vi "StartCSMs.vi"(8 "error in":errorcluster, 11 "Array":T1(array[cluster])=[{"prototype"="Normal-CSM.vi", "name"="Normal", "num"=1, "index"=0}, {"prototype"="Normal-CSM.vi", "name"=".SysLevel", "num"=1, "index"=0}, {"prototype"="Normal-CSM.vi", "name"="Normal.SubModule", "num"=1, "index"=0}, {"prototype"="Normal-CSM.vi", "name"="Normal2", "num"=1, "index"=0}, {"prototype"="Normal-CSM.vi", "name"=".SysLevel2", "num"=1, "index"=0}, {"prototype"="Normal-CSM.vi", "name"="Normal.SubModule2", "num"=1, "index"=0}, {"prototype"="Normal-CSM.vi", "name"="worker", "num"=3, "index"=0}, {"prototype"="Normal-CSM.vi", "name"="worker2", "num"=3, "index"=0}, {"prototype"="Chain1.vi", "name"="Chain", "num"=1, "index"=1}, {"prototype"="Chain2.vi", "name"="Chain", "num"=1, "index"=2}, {"prototype"="Chain3.vi", "name"="Chain", "num"=1, "index"=3}, {"prototype"="CSM\\CSM-Testcase.lvlibp\\testcases\\CSM\\Normal-CSM.vi", "name"="lvlibp", "num"=1, "index"=0}, {"prototype"="CSM\\CSM-Testcase2.lvlibp\\testcases\\CSM\\Normal-CSM.vi", "name"="lvlibp2", "num"=1, "index"=0}]) -> (0 "error out":errorcluster, 2 "CSMs":string[](array[string]))   [LabVIEW 2017]
uses:
  src/user.lib/_NEVSTOP/Communicable State Machine(CSM)/Communicable State Machine.lvlib
  src/user.lib/_NEVSTOP/Communicable State Machine(CSM)/_Shared/CSM Shared.lvlib
panel:
  out "Waited (ms)":u32
  out "CSMs Left":string[](array[string])
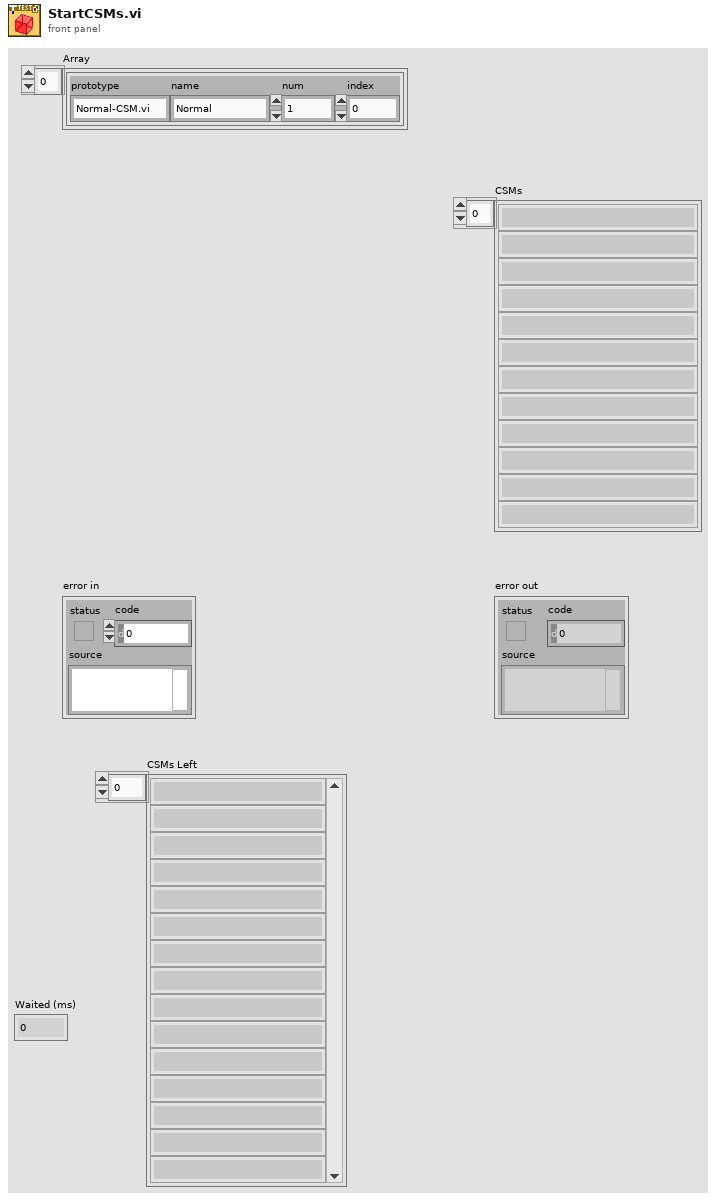
[diagram p1: front panel]
types:
  T1 = cluster{"prototype":string, "name":string, "num":i32, "index":i32}[]
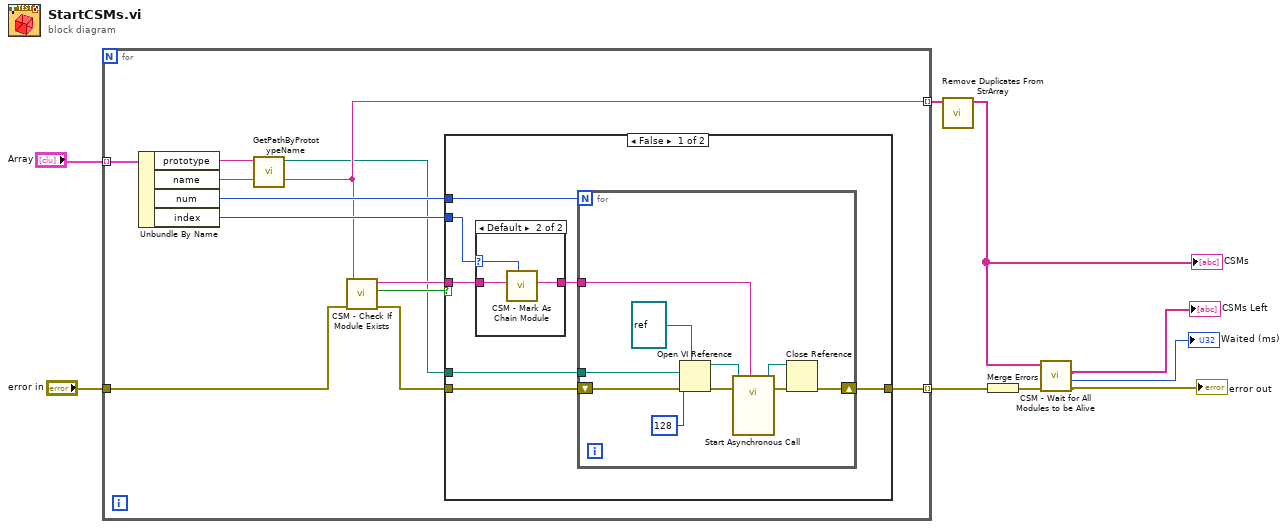
[diagram p0: block diagram]
diagram:
  n1 = for {
    tunnel: [w20] -> w6 mode=indexing
    tunnel: "Array" -> [w16] mode=indexing
    tunnel: "error in" -> [w15]
    tunnel: [w12] -> w7 mode=indexing
    n2 = Unbundle By Name(w16) -> ("prototype"=w11:string, "name"=w12:string, "num"=w14:i32, "index"=w13:i32)
    n3 = call "GetPathByPrototypeName.vi"("prototype"=w11) -> ("path"=w10:path)  [unwired: 10 in]
    n4 = call "CSM - Check If Module Exists.vi"("Error In"=w15, "CSM Name"=w12) -> ("error out"=w19:errorcluster, "Exist?"=w17:bool, "CSM Name (Dup)"=w18:string)  [unwired: 7 in]
    n5 = case shown="False" w17 {
      tunnel: [w27 w42] -> w20
      tunnel: w19 -> [w26 w42]
      tunnel: w18 -> [w23 _]
      tunnel: w14 -> [w25 _]
      tunnel: w13 -> [w24 _]
      tunnel: w10 -> [w21 _]
      frame False {
        n6 = case shown="Default" w24 {
          selector: w24 -> [_ w31]
          tunnel: w23 -> [w28 w30]
          tunnel: [w28 w29] -> w22
          frame 0 {
          }
          frame Default {
            n7 = call "CSM - Mark As Chain Module.vi"("Order"=w31, "CSM Name"=w30) -> ("CSM Name (Marked As Chain)"=w29:string)  [unwired: 8 in]
          }
        }
        n8 = for {
          N: w25 -> [_]
          tunnel: w22 -> [w35]
          shift-right: [w36] -> w27
          shift-left: w26 -> [w33]
          tunnel: w21 -> [w32]
          n9 = Open VI Reference(type specifier VI Refnum (for type only)=refnum<vi> refnum, vi path=w32, options=128, error in (no error)=w33) -> (vi reference=w38:refnum<vi>, error out=w40:errorcluster)  [unwired: 2 in]
          n10 = call-by-ref "Start Asynchronous Call"(reference=w38, error in=w40, "Name (\"\" to Use UUID)"=w35) -> (reference out=w37:refnum<vi>, error out=w39:errorcluster)  [unwired: 11 in]
          n11 = Close Reference(reference=w37, error in (no error)=w39) -> (error out=w36:errorcluster)
        }
      }
      frame True {
      }
    }
  }
  n12 = call "Remove Duplicates From StrArray.vi"("StrArray In"=w7) -> ("StrArray"=w1:string[])  [unwired: 9 in, 1 out]
  "CSMs" <- w1
  n13 = Merge Errors(w6) -> (w5:errorcluster)
  n14 = call "CSM - Wait for All Modules to be Alive.vi"("Error In"=w5, "CSM Names"=w1) -> ("error out"=→"error out":errorcluster, "Waited (ms)"=→"Waited (ms)":u32, "CSMs Left"=→"CSMs Left":string[])  [unwired: 7 in]
